vi "Get Created Queues.vi"(10 "Queue Mailbox":refnum<data-value>) -> (0 "error out":errorcluster, 2 "Created Queues":map{string, refnum<data-value>}(c390))   [LabVIEW 2021, in "jettl.lvlib" / "Queue Mailbox.lvlib"]
uses:
  Queue Mailbox.lvlib
  Queue Mailbox/Queue Mailbox.lvclass
  Msg Strategy/Msg Strategy.lvclass
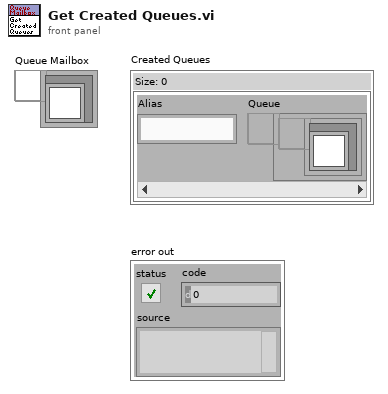
[diagram p1: front panel]
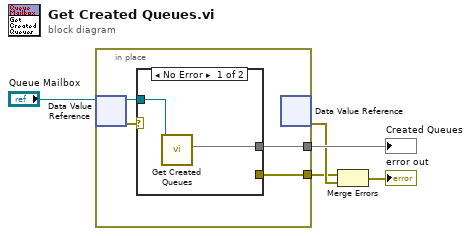
[diagram p0: block diagram]
diagram:
  n1 = in-place {
    in-place-border: [w9] -> w1
    in-place-border: [w8] -> w3
    n2 = in-place-dvr #1("Queue Mailbox") -> (w6:refnum<class "Queue Mailbox.lvclass">, w7:errorcluster)
    n3 = case shown="No Error" w7 {
      selector: w7 -> [_ w12]
      tunnel: w6 -> [w11 _]
      tunnel: [_ w12] -> w9
      tunnel: [w10 _] -> w8
      frame No Error {
        n4 = call "Get Created Queues.vi"("Queue Mailbox in"=w11) -> ("Created Queues"=w10:map{string, refnum<data-value>})  [unwired: 10 in]
      }
      frame Error {
      }
    }
    n5 = in-place-dvr #1() -> (w2:errorcluster)  [unwired: 1 in, 1 out]
  }
  "Created Queues" <- w3
  n6 = Merge Errors(w1, w2) -> (→"error out":errorcluster)
